vi "Set Name.vi"(7 "Unique ID":string, 8 "error in (no error)":errorcluster, 10 "Name":string, 11 "Test Executive in":refnum<class "Test Executive.lvclass">) -> (0 "error out":errorcluster, 3 "Test Executive out":refnum<class "Test Executive.lvclass">)   [LabVIEW 2019, in "Test Executive.lvlib" / "Test Executive.lvclass"]
uses:
  <vilib>/gpm_packages/@cs/test-executive/Source/Test Executive/TestExecutive/Test Executive.lvclass
  <vilib>/gpm_packages/@cs/test-executive/Source/Test Executive/TestExecutive/Test Executive.lvclass/Test Executive.ctl
  <vilib>/gpm_packages/@cs/linked-list/Source/Linked List/Linked List Ref/Linked List Ref.lvclass
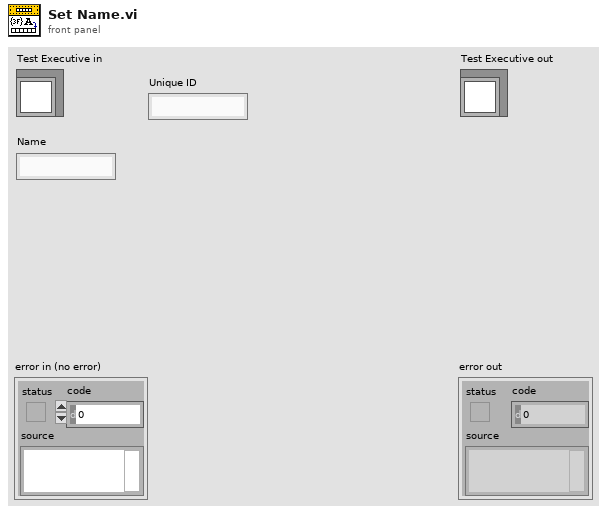
[diagram p1: front panel]
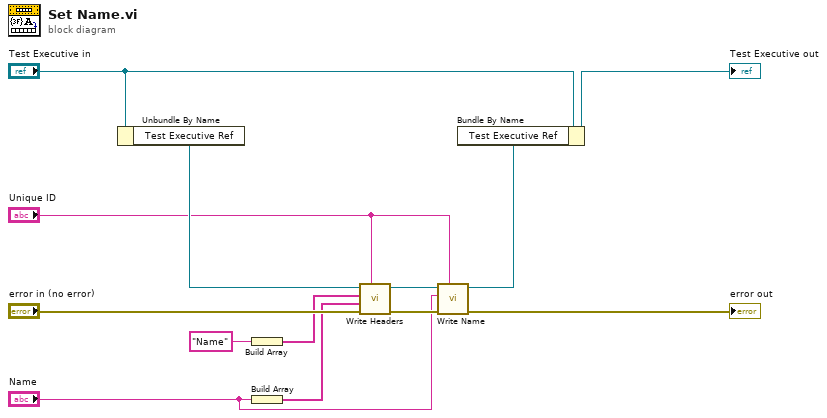
[diagram p0: block diagram]
diagram:
  n1 = Unbundle By Name("Test Executive in") -> ("Test Executive Ref"=w10:refnum<data-value>)
  n2 = Build Array("Name") -> (w8:string[])
  n3 = Build Array("Name") -> (w7:string[])
  n4 = call <vilib>:"Write Headers.vi"("Linked List ID"="Unique ID", "error in (no error)"="error in (no error)", "Header Values"=w7, "Header Names"=w8, "Linked List Ref"=w10) -> ("error out"=w6:errorcluster, "Linked List Ref out"=w5:refnum<data-value>)  [unwired: 5 in]
  n5 = call <vilib>:"Write Name.vi"("Linked List ID"="Unique ID", "error in (no error)"=w6, "Name"="Name", "Linked List Ref"=w5) -> ("error out"=→"error out":errorcluster, "Linked List Ref out"=w2:refnum<data-value>)  [unwired: 6 in]
  n6 = Bundle By Name(cluster="Test Executive in", "Test Executive Ref"=w2) -> (→"Test Executive out":refnum<class "Test Executive.lvclass">)
